vi "Auton_Sc_Shoot_Move.vi"   [LabVIEW 2019]
uses:
  Robot Global Data.vi
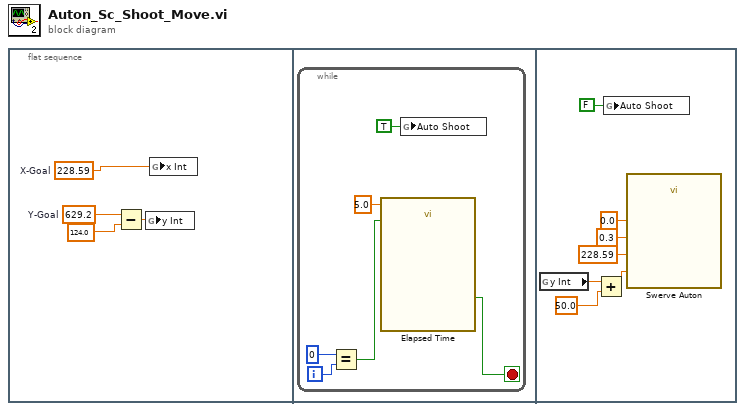
[diagram p0: block diagram]
diagram:
  n1 = flat-sequence {
    frame #0 {
      w4 = 228.59  # X-Goal
      w2 = 629.2  # Y-Goal
      n2 = Subtract(x=w2, y=124.0) -> (x-y=w3:dbl)
      n3 = global write "Robot Global Data.vi" "y Int"(w3) -> ()
      n4 = global write "Robot Global Data.vi" "x Int"(w4) -> ()
    }
    frame #1 {
      n5 = while {
        i -> [w6]
        stop <- w9 stop-if-true
        n6 = Equal?(x=0, y=w6) -> (x = y?=w5:bool)
        n7 = call "Elapsed Time"("Time Target (s)"=5.0, "Reset"=w5) -> ("Time has Elapsed"=w9:bool)  [unwired: 10 in, 7 out]
        n8 = global write "Robot Global Data.vi" "Auto Shoot"(TRUE ("Auto Shoot")) -> ()
      }
    }
    frame #2 {
      n9 = global read "Robot Global Data.vi" "y Int"() -> (w13:dbl)
      n10 = Add(x=w13, y=50.0 ("y Distance")) -> (x+y=w12:dbl)
      n11 = global write "Robot Global Data.vi" "Auto Shoot"(FALSE ("Auto Shoot")) -> ()
      n12 = call "Swerve Auton.vi"("Heading"=0.0, "y Distance"=w12, "x Distance"=228.59, "Power"=0.3) -> ()  [unwired: 8 in]
    }
  }
